vi "zmq_connect.vi"(3 "error in":errorcluster, 4 "endpoint":string, 5 "socket in":refnum<class "zmq_socket.lvclass">) -> (0 "error out":errorcluster, 2 "socket out":refnum<class "zmq_socket.lvclass">)   [LabVIEW 2020, in "zeromq.lvlib" / "zmq_socket.lvclass"]
doc: "Attempt to connect the socket created with zmq_socket to the given <b>endpoint</b>. The endpoint string should specify the protocol, host and port for the connection, e.g.\n tcp://localhost:1234\n inproc://namedprocess\n\nNote that unlike regular TCP sockets, you can connect to a host without the host having bound the port first.\n\nDetailed API documentation: http://api.zeromq.org/3-2:zmq-connect"
uses:
  zmq_socket.lvclass
  zmq_socket.lvclass/zmq_socket.ctl
  Error Cluster From Error Code.vi
  zeromq.lvlib
panel:
  # "ØMQ"
  # "labview"
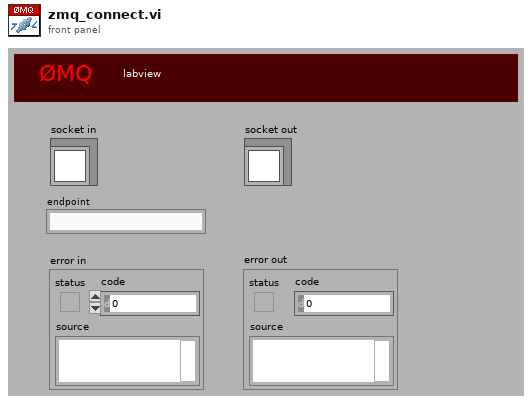
[diagram p1: front panel]
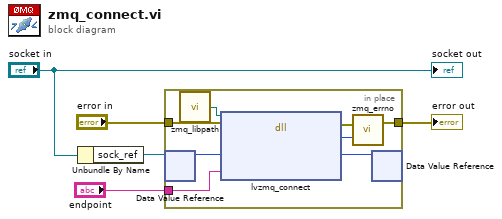
[diagram p0: block diagram]
diagram:
  n1 = Unbundle By Name("socket in") -> ("sock_ref"=w1:refnum<data-value>)
  n2 = in-place {
    in-place-border: "endpoint" -> [w13]
    in-place-border: "error in" -> [w12]
    in-place-border: [w9] -> w3
    n3 = in-place-dvr #1(w1) -> (w8:u64)  [unwired: 1 out]
    n4 = call "zmq_libpath.vi"() -> ("path"=w6:path)
    n5 = dll-call lib="?" fn="lvzmq_connect"(path in=w6, error in=w12, "sock_obj"=w8, "endpoint"=w13) -> (error out=w11:errorcluster, "return type"=w10:i32, "sock_obj"=w7:u64)  [unwired: 2 in, 1 out]
    n6 = call "zmq_errno.vi"("retval"=w10, "error in"=w11) -> ("error out"=w9:errorcluster)  [unwired: 1 out]
    n7 = in-place-dvr #1(w7) -> ()  [unwired: 2 out]
  }
  "error out" <- w3
  "socket out" <- "socket in"
